vi "Lake Shore 335 Configure Input Parameters.vi"(0 "VISA resource name":refnum<visa-resource-name>="GPIB0::12::INSTR") -> ()   [LabVIEW 2017]
doc: "This VI was designed to demonstrate typical usage of sub VIs containing the more common 335 functions. The VI Initializes the instrument, allows the user to determine if heater output control parameters and setpoint values are sent, takes a single sensor reading, and then closes the instrument."
uses:
  <instrlib>/Lake Shore 335/Public/Data/Sensor Data (Single Reading).vi
  <instrlib>/Lake Shore 335/Lake Shore 335.lvlib
panel:
  in  "Configure Input Parameters (0: Don't Configure)":u16(ring) items=["Don't Configure", "Configure"]
  in  "Temperature Limit (0)":u16=335
  in  "Enable \nCompensation (F: Off)":bool
  in  "Curve (0:None)":u16(ring)=21 items=["None"=0, "DT-470"=1, "DT-670"=2, "DT-500-D"=3, "DT-500-E1"=4, "PT-100"=6, "PT-1000"=7, "RX-102A-AA"=8, "RX-202A-AA"=9, "Type K"=12, "Type E"=13, "Type T"=14, "AuFe 0.03%"=15, "AuFe 0.07%"=16, "User 21"=21, "User 22"=22, "User 23"=23, "User 24"=24, "User 25"=25, "User 26"=26, "User 27"=27, "User 28"=28, "User 29"=29, "User 30"=30, "User 31"=31, "User 32"=32, "User 33"=33, "User 34"=34, "User 35"=35, "User 36"=36, "User 37"=37, "User 38"=38, "User 39"=39, "User 40"=40, "User 41"=41, "User 42"=42, "User 43"=43, "User 44"=44, "User 45"=45, "User 46"=46, "User 47"=47, "User 48"=48, "User 49"=49, "User 50"=50, "User 51"=51, "User 52"=52, "User 53"=53, "User 54"=54, "User 55"=55, "User 56"=56, "User 57"=57, "User 58"=58, "User 59"=59]
  in  "Preferred Units (1:Kelvin)":u16(ring)=1 items=["Kelvin"=1, "Celsius"=2, "Sensor Units"=3]
  in  "Diode Current (0:10 uA)":u16(ring) items=["10 uA", "1 mA"]
  in  "Sensor Type and Range (0:Disabled)":u16(ring)=11 items=["Disabled", "Diode 2.5 V (Silicon)", "Diode 10 V (GaAlAs)", "PTC RTD Autorange", "PTC RTD 10 Ohm", "PTC RTD 30 Ohm", "PTC RTD 100 Ohm", "PTC RTD 300 Ohm", "PTC RTD 1 kOhm", "PTC RTD 3 kOhm", "PTC RTD 10 kOhm", "NTC RTD Autorange", "NTC RTD 10 Ohm", "NTC RTD 30 Ohm", "NTC RTD 100 Ohm", "NTC RTD 300 Ohm", "NTC RTD 1 kOhm", "NTC RTD 3 kOhm", "NTC RTD 10 kOhm", "NTC RTD 30 kOhm", "NTC RTD 100 kOhm", "Thermocouple"]
  in  "Input (0:A)":u16(ring) items=["A", "B"]
  in  "Input Name (\"\")":string="miSensor"
  in  "Polarity (0:Unipolar)":u16(ring) items=["Unipolar", "Bipolar"]
  in  "Output Type (0:Current)":u16(ring) items=["Current", "Voltage"]
  in  "Heater Output (1:1)":u16(ring)=1 items=["1"=1, "2"=2]
  in  "Heater Resistance (1:25 Ohm)":u16(ring)=2 items=["25 Ohm"=1, "50 Ohm"=2]
  in  "Max User Current (1.732)":dbl=1.732 format="%.3f"
  in  "Heater Out Display (1:Current)":u16(ring)=1 items=["Current"=1, "Power"=2]
  in  "Max Current (0:User Specified)":u16(ring)=2 items=["User Specified", "0.707 A", "1.0 A", "1.141 A", "1.732 A"]
  in  "Mode (0:Off)":u16(ring)=1 items=["Off", "Closed Loop PID", "Zone", "Open Loop", "Monitor Out", "Warmup Supply"]
  in  "Power Up Enable (F: Off)":bool
  in  "Input (0:None)":u16(ring)=1 items=["None", "A", "B"]
  in  "Input (0:A)":u16(ring) items=["A", "B"]
  in  "Data Source (0:Kelvin)":u16(ring) items=["Kelvin", "Celsius", "Sensor Units"]
  out "Sensor Data":dbl format="%.4f"
  in  "Configure Setpoint (0: Don't Configure)":u16(ring) items=["Don't Configure", "Configure"]
  in  "Setpoint (0.0000)":dbl format="%.4f"
  in  "Manual Output (0.00 %)":dbl format="%.2f"
  in  "Range (0:Off)":u16(ring) items=["Off", "Low (On)", "Medium", "High"]
  in  "Rate (D) (0.0 %)":dbl format="%.1f"
  in  "Reset (I) (20.0)":dbl=20.0 format="%.1f"
  in  "Gain (P) (50.0)":dbl=50.0 format="%.1f"
  in  "Serial Configuration":T1={"Baud Rate"=57600, "Parity"=1, "Data Bits"=7, "Stop Bits"=10, "Flow Control"=0} {"Flow Control" items=["None", "XON/XOFF", "RTS/CTS", "XON/XOFF & RTS/CTS", "DTR/DSR", "XON/XOFF & DTR/DSR"]; "Stop Bits" items=["1.0"=10, "1.5"=15, "2.0"=20]; "Data Bits" items=["7"=7, "8"=8]; "Parity" items=["None", "Odd", "Even", "Mark", "Space"]; "Baud Rate" items=["300"=300, "600"=600, "1200"=1200, "2400"=2400, "4800"=4800, "9600"=9600, "19200"=19200, "38400"=38400, "57600"=57600]}
  in  "Configure Control Parameters (0: Don't Configure)":u16(ring) items=["Don't Configure", "Configure"]
  # "(c) 2011 Lake Shore Cryotronics Inc.  ALL RIGHTS RESERVED."
  # "(c) 2020 SIE.SAI MODIFICADO.  ALL RIGHTS RESERVED."
  # "Input Parameters"
  # "Output Control Parameters"
  # "Output Setpoint"
  # "Sensor Data"
  # "Settings for Either Heater Output"
  # "Settings for Heater Output 2 Only"
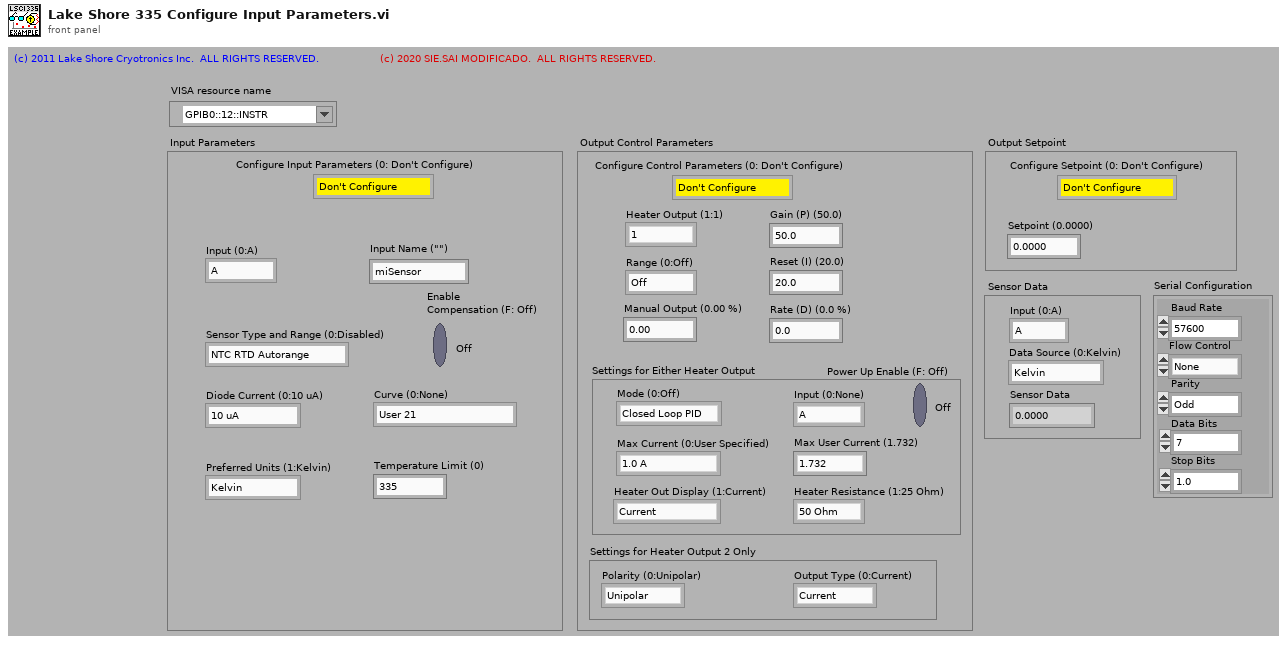
[diagram p1: front panel]
types:
  T1 = cluster{"Baud Rate":u32, "Parity":u16, "Data Bits":u16, "Stop Bits":u16, "Flow Control":u16}
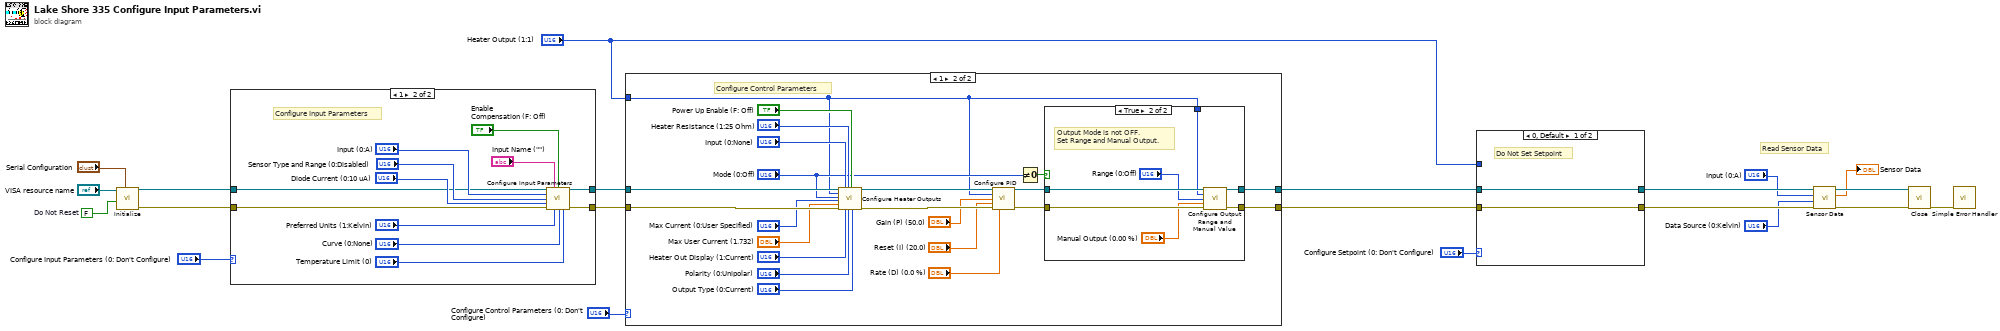
[diagram p0: block diagram]
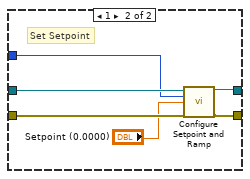
[diagram p3: hidden frame]
diagram:
  w16 = FALSE  # Do Not Reset
  # "Read Sensor Data"
  n1 = call <instrlib>:"Initialize.vi"("Serial Configuration"="Serial Configuration", "Reset (True)"=w16, "VISA resource name"="VISA resource name") -> ("error out"=w4:errorcluster, "VISA resource name out"=w2:refnum<visa-resource-name>)  [unwired: 7 in]
  n2 = case shown="1" "Configure Input Parameters (0: Don't Configure)" {
    tunnel: w2 -> [w23 w27]
    tunnel: w4 -> [w22 w26]
    tunnel: [w22 w25] -> w3
    tunnel: [w23 w24] -> w1
    frame 0, Default {
      # "Do Not Configure Input Parameters"
    }
    frame 1 {
      # "Configure Input Parameters"
      n3 = call <instrlib>:"Configure Input Parameters.vi"("VISA resource name"=w27, "Input Name (\"\")"="Input Name (\"\")", "Enable \nCompensation (F: Off)"="Enable \nCompensation (F: Off)", "Input (0:A)"="Input (0:A)", "Sensor Type and Range (0:Disabled)"="Sensor Type and Range (0:Disabled)", "Diode Current (0:10 uA)"="Diode Current (0:10 uA)", "error in (no error)"=w26, "Preferred Units (1:Kelvin)"="Preferred Units (1:Kelvin)", "Curve (0:None)"="Curve (0:None)", "Temperature Limit (0)"="Temperature Limit (0)") -> ("VISA resource name out"=w24:refnum<visa-resource-name>, "error out"=w25:errorcluster)  [unwired: 4 in]
    }
  }
  n4 = case shown="1" "Configure Control Parameters (0: Don't Configure)" {
    tunnel: "Heater Output (1:1)" -> [_ w38]
    tunnel: w1 -> [w37 w53]
    tunnel: w3 -> [w36 w52]
    tunnel: [w36 w57] -> w17
    tunnel: [w37 w56] -> w18
    frame 0, Default {
      # "Do Not Configure Control Parameters"
    }
    frame 1 {
      # "Configure Control Parameters"
      n5 = call <instrlib>:"Configure Heater Outputs.vi"("VISA resource name"=w53, "Heater Output (1:1)"=w38, "Mode (0:Off)"="Mode (0:Off)", "Max Current (0:User Specified)"="Max Current (0:User Specified)", "Max User Current (1.732)"="Max User Current (1.732)", "error in (no error)"=w52, "Input (0:None)"="Input (0:None)", "Heater Out Display (1:Current)"="Heater Out Display (1:Current)", "Heater Resistance (1:25 Ohm)"="Heater Resistance (1:25 Ohm)", "Polarity (0:Unipolar)"="Polarity (0:Unipolar)", "Power Up Enable (F: Off)"="Power Up Enable (F: Off)", "Output Type (0:Current)"="Output Type (0:Current)") -> ("VISA resource name out"=w55:refnum<visa-resource-name>, "error out"=w54:errorcluster)  [unwired: 6 in]
      n6 = call <instrlib>:"Configure PID.vi"("VISA resource name"=w55, "Output's Control Loop (1:1)"=w38, "Gain (P) (50.0)"="Gain (P) (50.0)", "Reset (I) (20.0)"="Reset (I) (20.0)", "error in (no error)"=w54, "Rate (D) (0.0 %)"="Rate (D) (0.0 %)") -> ("VISA resource name out"=w59:refnum<visa-resource-name>, "error out"=w58:errorcluster)  [unwired: 8 in]
      n7 = Not Equal To 0?(x="Mode (0:Off)") -> (x != 0?=w48:bool)
      n8 = case shown="True" w48 {
        tunnel: w59 -> [w61 w68]
        tunnel: w58 -> [w60 w67]
        tunnel: [w60 w66] -> w57
        tunnel: [w61 w65] -> w56
        tunnel: w38 -> [_ w64]
        frame False {
          # "Output Mode is OFF.  Do not\nset Range and Manual Output (prevents \nExecution Error)."
        }
        frame True {
          # "Output Mode is not OFF.\nSet Range and Manual Output."
          n9 = call <instrlib>:"Configure Output Range and Manual Value.vi"("VISA resource name"=w68, "Heater Output (1:1)"=w64, "Range (0:Off)"="Range (0:Off)", "Manual Output (0.00 %)"="Manual Output (0.00 %)", "error in (no error)"=w67) -> ("VISA resource name out"=w65:refnum<visa-resource-name>, "error out"=w66:errorcluster)  [unwired: 9 in]
        }
      }
    }
  }
  n10 = case shown="0, Default" "Configure Setpoint (0: Don't Configure)" {
    tunnel: "Heater Output (1:1)" -> [_ w74]
    tunnel: w18 -> [w70 w75]
    tunnel: w17 -> [w69 w76]
    tunnel: [w69 w72] -> w13
    tunnel: [w70 w73] -> w14
    frame 0, Default {
      # "Do Not Set Setpoint"
    }
    frame 1 {
      # "Set Setpoint"
      n11 = call <instrlib>:"Configure Setpoint and Ramp.vi"("VISA resource name"=w75, "Output's Control Loop (1:1)"=w74, "Setpoint (0.0000)"="Setpoint (0.0000)", "error in (no error)"=w76) -> ("VISA resource name out"=w73:refnum<visa-resource-name>, "error out"=w72:errorcluster)  [unwired: 10 in]
    }
  }
  n12 = call-poly <instrlib>:"Sensor Data.vi"("error in (no error)"=w13, "Data Source (0:Kelvin)"="Data Source (0:Kelvin)", "Input (0:A)"="Input (0:A)", "VISA resource name"=w14) -> ("error out"=w11:errorcluster, "Sensor Data"=→"Sensor Data":dbl, "VISA resource name out"=w12:refnum<visa-resource-name>)  [unwired: 5 in]
  n13 = call <instrlib>:"Close.vi"("error in (no error)"=w11, "VISA resource name"=w12) -> ("error out"=w19:errorcluster)  [unwired: 9 in]
  n14 = call <vilib>:"Simple Error Handler.vi"("error in (no error)"=w19) -> ()  [unwired: 4 in, 5 out]
